vi "Finite Buffered Acquisition with Analysis.vi"() -> ()   [LabVIEW 2009]
uses:
  <vilib>/DAQmx/read.llb/DAQmx Read (Analog Wfm 1Chan NSamp).vi
  <vilib>/DAQmx/configure/timing.llb/DAQmx Timing (Sample Clock).vi
  <vilib>/DAQmx/create/channels.llb/DAQmx Create Channel (AI-Voltage-Basic).vi
panel:
  out "Positive Peak":dbl
  out "Negative Peak":dbl
  in  "samples per channel":i32=1000
  in  "rate":dbl=1000.0 format="%0.2f"
  in  "physical channels":tag
  out "Acquired Data":waveform(dbl)(graph)
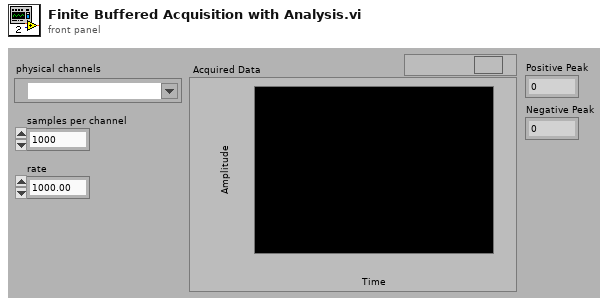
[diagram p1: front panel]
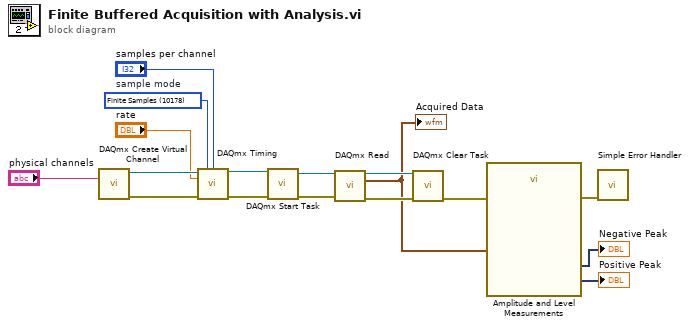
[diagram p0: block diagram]
diagram:
  w9 = 10178 items=["Finite Samples"=10178, "Continuous Samples"=10123]  # sample mode
  n1 = call-poly <vilib>:"DAQmx Create Virtual Channel.vi"("physical channels"="physical channels") -> ("task out"=w8:refnum<k21>, "error out"=w7:errorcluster)  [unwired: 13 in]
  n2 = call-poly <vilib>:"DAQmx Timing.vi"("task/channels in"=w8, "sample mode"=w9, "samples per channel"="samples per channel", "rate"="rate", "error in"=w7) -> ("task out"=w11:refnum<k21>, "error out"=w10:errorcluster)  [unwired: 9 in]
  n3 = call <vilib>:"DAQmx Start Task.vi"("task/channels in"=w11, "error in"=w10) -> ("task out"=w12:refnum<k21>, "error out"=w13:errorcluster)  [unwired: 12 in]
  n4 = call-poly <vilib>:"DAQmx Read.vi"("task/channels in"=w12, "error in"=w13) -> ("task out"=w3:refnum<k21>, "data"=w1:waveform(dbl), "error out"=w2:errorcluster)  [unwired: 11 in]
  "Acquired Data" <- w1
  n5 = call <vilib>:"DAQmx Clear Task.vi"("task in"=w3, "error in"=w2) -> ("error out"=w17:errorcluster)  [unwired: 13 in]
  n6 = call "Amplitude and Level Measurements"("Signals"=w1, "error in (no error)"=w17) -> ("Negative Peak"=→"Negative Peak":dynamicdata, "Positive Peak"=→"Positive Peak":dynamicdata, "error out"=w16:errorcluster)  [unwired: 11 in]
  n7 = call <vilib>:"Simple Error Handler.vi"("error in (no error)"=w16) -> ()  [unwired: 4 in, 5 out]
